vi "daq.vi"() -> ()   [LabVIEW 2020]
uses:
  <vilib>/DAQmx/read.llb/DAQmx Read (Digital 1D Bool 1Chan 1Samp).vi
  <vilib>/DAQmx/create/channels.llb/DAQmx Create Channel (DI-Digital Input).vi
  <vilib>/DAQmx/miscellaneous.llb/DAQmx Fill In Error Info.vi
panel:
  in  "stop":bool
  out "ErrOut":errorcluster
  in  "ErrIn":errorcluster
  out "Array":bool[](array[boolean])
  in  "Chanels":tag="Dev1/port0"
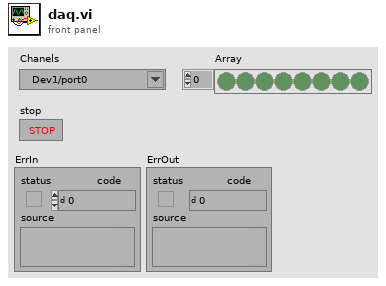
[diagram p1: front panel]
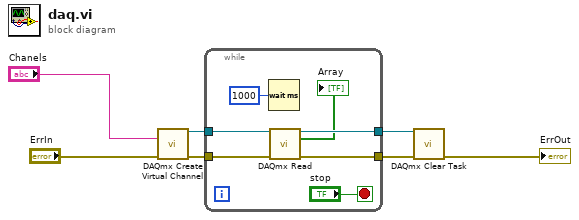
[diagram p0: block diagram]
diagram:
  n1 = call-poly <vilib>:"DAQmx Create Virtual Channel.vi"("lines"="Chanels", "error in"="ErrIn") -> ("task out"=w7:refnum<k21>, "error out"=w6:errorcluster)  [unwired: 12 in]
  n2 = while {
    tunnel: w6 -> [w14]
    tunnel: [w12] -> w4
    tunnel: w7 -> [w8]
    tunnel: [w13] -> w5
    stop <- "stop" stop-if-true
    n3 = Wait (ms)(milliseconds to wait=u32 1000) -> ()  [unwired: 1 out]
    n4 = call-poly <vilib>:"DAQmx Read.vi"("task/channels in"=w8, "error in"=w14) -> ("task out"=w13:refnum<k21>, "data"=→"Array":bool[], "error out"=w12:errorcluster)  [unwired: 11 in]
  }
  n5 = call <vilib>:"DAQmx Clear Task.vi"("task in"=w5, "error in"=w4) -> ("error out"=→"ErrOut":errorcluster)  [unwired: 13 in]
